vi "_MainOpenMV_New.vi"() -> (2 "Script Out":string)   [LabVIEW 2016]
uses:
  VIs/_subs/CameraSetup.ctl
panel:
  in  "Make Main":bool
  out "ROI":T1={"left"=0, "top"=0, "right"=320, "bottom"=240}
  in  "Set ROI":bool
  out "roi":string
  in  "Set Threshold":bool
  in  "clear":bool
  out "Plots":T2
  out "Lab":string="[10,90,-40,40,-40,40]"
  out "Tx Buffer":string
  in  "Play":bool
  in  "Serial Port":refnum<visa-resource-name>="ASRL30::INSTR"
  out "Version":string
  in  "Connect":bool
  out "FPS":dbl format="%#.2g"
  in  "Tabs":enum32{"Simple View", "REPL", "Python"}(tab)
  in  "Destination Info":enum32{"None", "UART", "SPI", "I2C", "WiFi"}(tab)
  in  "WiFi Info":T3={"WiFi"={"SSID"="", "Key"=""}, "SystemLink"={"APIKey"="", "Tag"="", "Type"="STRING"}}
  in  "Destination":enum16{"None", "UART", "SPI", "I2C", "WiFi"}(ring)
  out "Value":dbl(graph)
  in  "View":T4(ring)
  in  "Params":T5(tab)
  in  "Color Statistic":u16(ring) items=["l_mean", "l_median", "l_mode", "l_sdev", "l_min", "l_max", "l_lower quartile", "l_upper quartile", "a_mean", "a_median", "a_mode", "a_sdev", "a_min", "a_max", "a_lq", "a_uq", "b_mean", "b_median", "b_mode", "b_sdev", "b_max", "b_min", "b_lq", "b_uq", "All statistics"]
  in  "Gray Statistic":u16(ring)=1 items=["mean", "median", "mode", "sdev", "min", "max", "lower quartile", "upper quartile", "All statistics"]
  in  "Blob Params":T6={"B[0]_Feature"=enum."# blobs", "Lab thresholds"="[10,90,-20,20,-20,20]", "Min Pixels"=100, "Min Area (box)"=100, "Merge"=TRUE, "Margin for merge"=10}
  in  "Face Parameter":u16(ring) items=["# faces", "All data"]
  in  "QR Return":u16(ring)=4 items=["x", "y", "w", "h", "payload", "version", "ecc_level", "mask", "data_type", "All data"]
  in  "Ctrl D":bool
  in  "Grab Script":bool
  in  "Line":u8(slide) scale=0.0..25.0
  in  "Send Line":bool
  out "Console":string
  in  "Notepad":string
  in  "Ctrl C":bool
  out "rows":string="  1\n  2\n  3\n  4\n  5\n  6\n  7\n  8\n  9\n 10\n 11\n 12\n 13\n 14\n 15\n 16\n 17\n 18\n 19\n 20\n 21\n"
  in  "Script":string="# Show Color - lmean\n\nimport sensor, image, time\n\nsensor.reset()\nsensor.set_pixformat(sensor.RGB565)\nsensor.set_framesize(sensor.QVGA)\nsensor.skip_frames(time = 2000)\n\nsensor.set_auto_gain(False)\nsensor.set_auto_whitebal(False) \n\nclock = time.clock()\n\n\n\nwhile(True):\n    clock.tick()\n    img = sensor.snapshot()\n    \n    print(img.statistics()[0])\n"
  in  "New":bool
  in  "Load":bool
  in  "Save":bool
  in  "File":path
  in  "startCode":string
  out "Size":string
  in  "stop":bool
  out "image":picture
  # "LabVIEW OpenMV"
  # "Note: i2c and SPI and WiFi are having issues"
  # "Use P4 for Tx and P5 for Rx and GND for ground\n\nDefault BAUD rate is 19200 - you can change this\nby editing the Python code (Python tab)"
  # "Use P0 for MOSI, P1 for MISO, P2 for SCLK, P3 for SS (active low)\n and GND for ground\n\nThe default is being an SPI slave - note that you can miss data\nin this mode"
  # "Use P4 for SCL and P5 for SDA and GND for ground\n\nThis runs as an i2c slave"
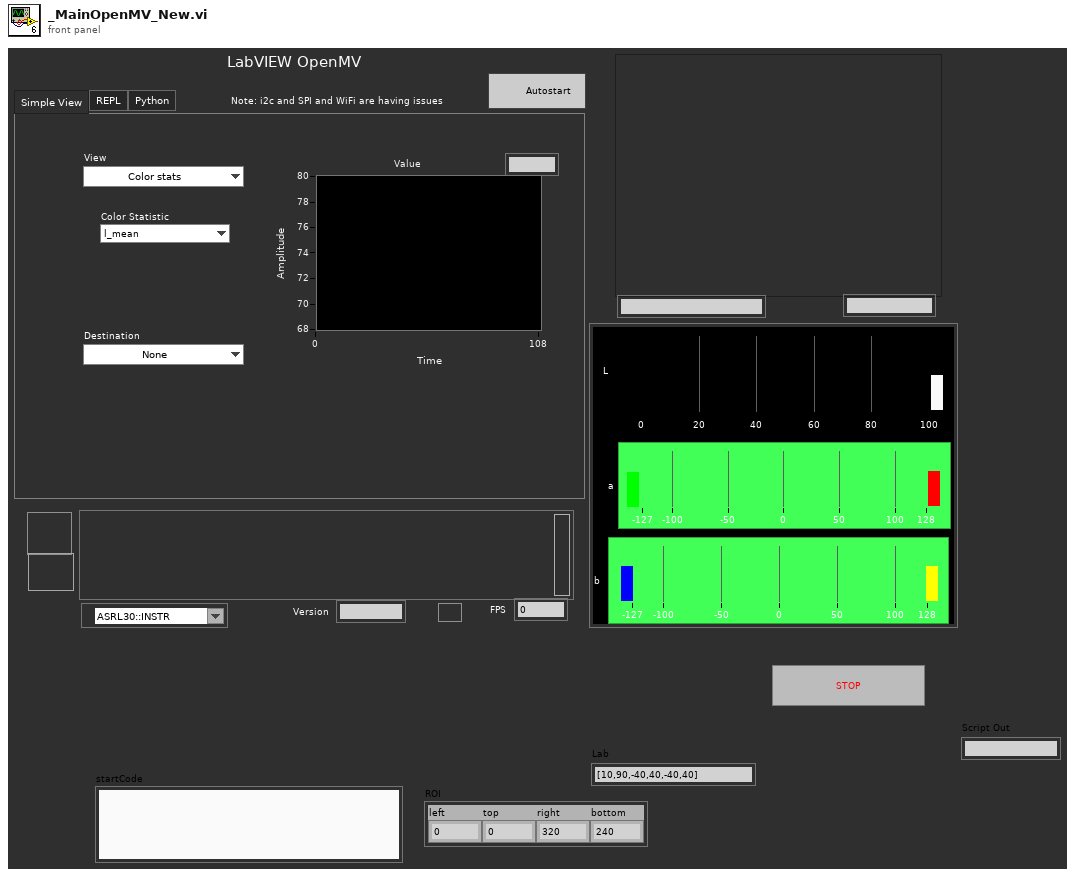
[diagram p1: front panel]
types:
  T1 = cluster{"left":i16, "top":i16, "right":i16, "bottom":i16}
  T2 = cluster{"L":dbl[], "a":cluster{i32, i32, dbl[]}, "b":cluster{i32, i32, dbl[]}}
  T3 = cluster{"WiFi":cluster{"SSID":string, "Key":string}, "SystemLink":cluster{"APIKey":string, "Tag":string, "Type":string}}
  T4 = enum16{"Color stats", "Greyscale stats", "Track Blobs", "Track Faces", "QRCode"}
  T5 = enum32{"C_ Stat", "G_Stats", "Blobs", "Face", "QR"}
  T6 = cluster{"B[0]_Feature":enum16{"x", "y", "width", "height", "pixels", "cx", "cy", "rotation", "code", "count", "# blobs", "All parameters"}, "Lab thresholds":string, "Min Pixels":i16, "Min Area (box)":i16, "Merge":bool, "Margin for merge":i16}
  T7 = enum8{"Enabled", "Disabled", "Disabled and Grayed Out"}
  T8 = typedef "CameraSetup.ctl" = cluster{"Format":enum16{"GRAYSCALE", "RGB565", "BAYER"}, "size":enum16{"QQQQVGA (40x30)", "QQQVGA (80x60)", "QQVGA (160x120)", "QVGA (320x240)", "VGA (640x480)", "LCD (128x160)", "B64x32 (64x32)", "B64x64", "B128x64", "B128x128"}, "Skip frames (ms)":u16, "autoGain":bool, "autoWhitebal":bool}
  T9 = typedef "imagedata.ctl" = cluster{"image type":i32, "image depth":i32, "image":u8[], "mask":u8[], "colors":u32[], "Rectangle":cluster{"left":i16, "top":i16, "right":i16, "bottom":i16}}
  T10 = cluster{"left":i32, "top":i32, "right":i32, "bottom":i32}
  T11 = typedef "eventvkey.ctl" = enum16{"ASCII", "Enter", "Return", "Shift", "Ctrl", "Alt", "Cmd", "Opt", "Caps", "NumLock", "Clear", "Break", "Up", "Down", "Left", "Right", "Insert", "Delete", "Home", "End", "PageUp", "PageDown", "Escape", "Help", "Pause", "ScrollLock", "F1", "F2", "F3", "F4", "F5", "F6", "F7", "F8", "F9", "F10", "F11", "F12", "F13", "F14", "F15", "F16", "F17", "F18", "F19", "F20", "F21", "F22", "F23", "F24", "Play", "VolumeUp", "VolumeDown", "Mute", "Two Byte Char"}
  T12 = cluster{"Shift":bool, "Ctrl":bool, "Alt":bool, "Cmd":bool, "Opt":bool}
  T13 = cluster{"Char":i16, "VKey":T11, "ScanCode":i16, "Mods":cluster{"Num Pad":bool, "Menu Key":bool}, "PlatMods":cluster{"Shift":bool, "Ctrl":bool, "Alt":bool, "Cmd":bool, "Opt":bool}, "FocusObj":refnum<vi>}
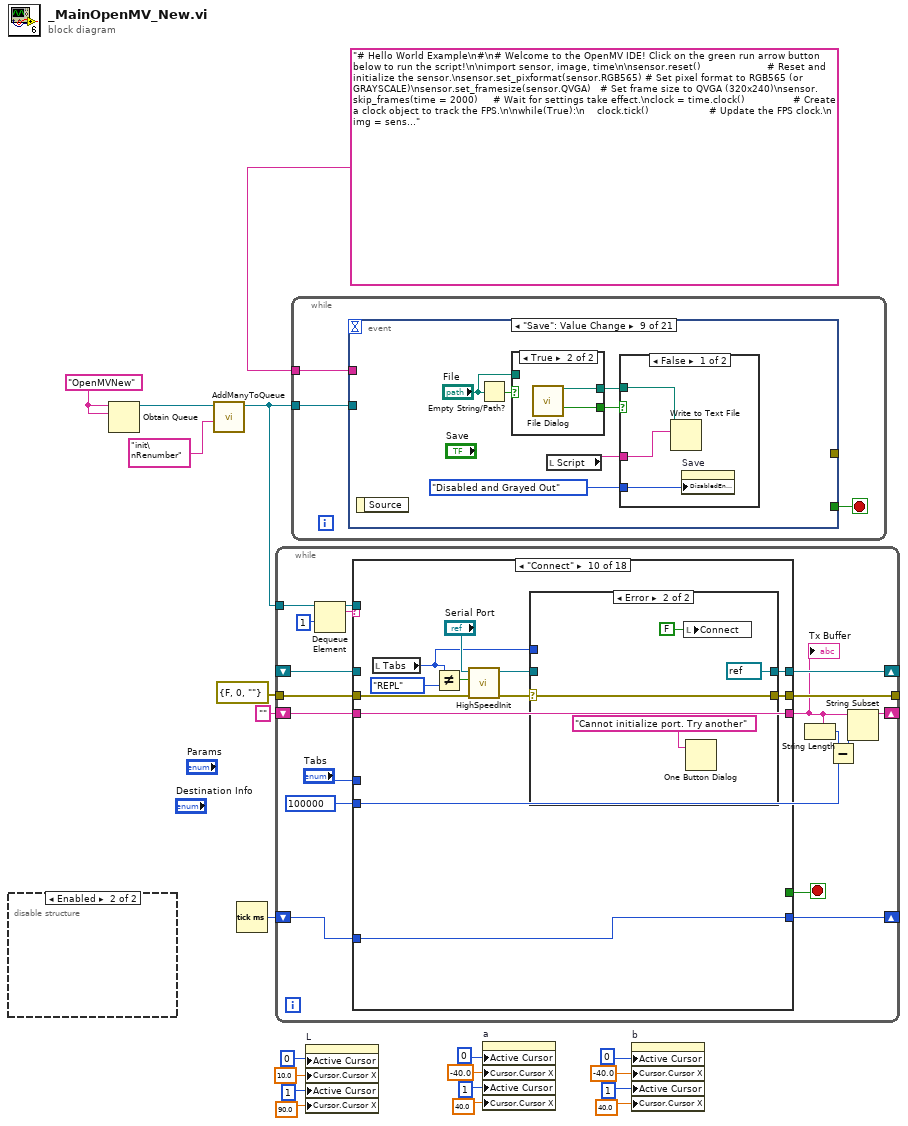
[diagram p0: block diagram]
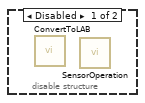
[diagram p2: hidden frame]
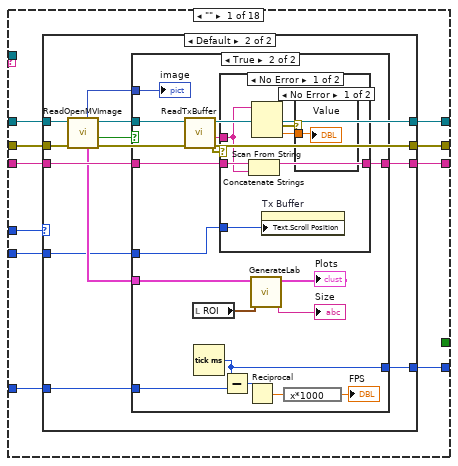
[diagram p3: hidden frame]
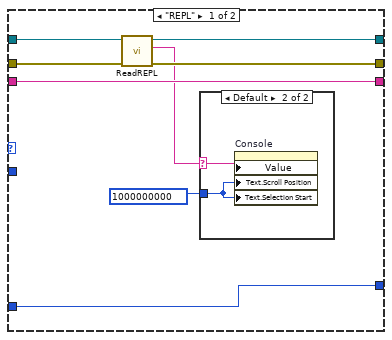
[diagram p4: hidden frame]
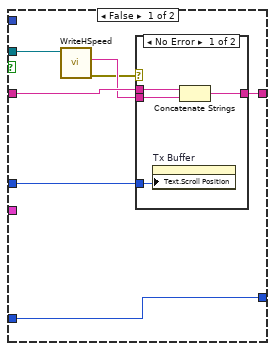
[diagram p6: hidden frame]
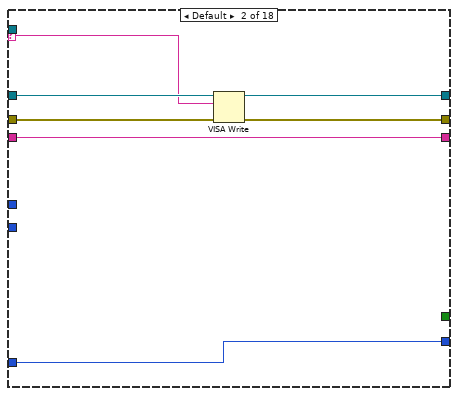
[diagram p10: hidden frame]
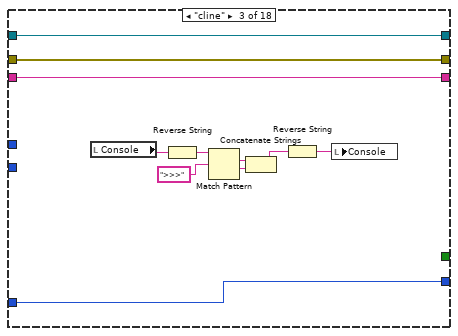
[diagram p11: hidden frame]
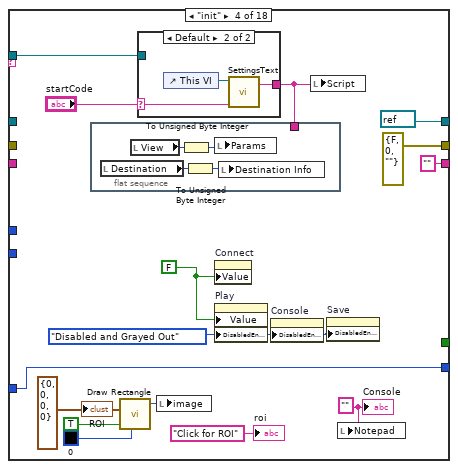
[diagram p12: hidden frame]
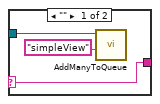
[diagram p13: hidden frame]
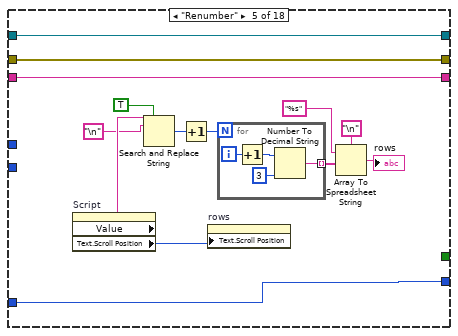
[diagram p14: hidden frame]
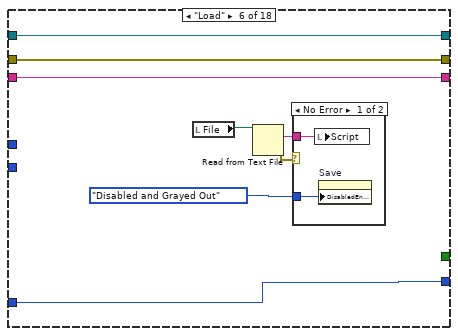
[diagram p15: hidden frame]
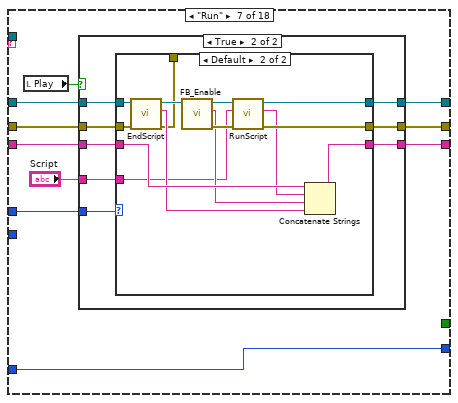
[diagram p17: hidden frame]
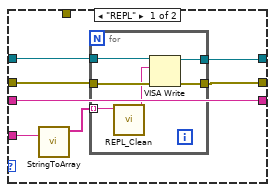
[diagram p19: hidden frame]
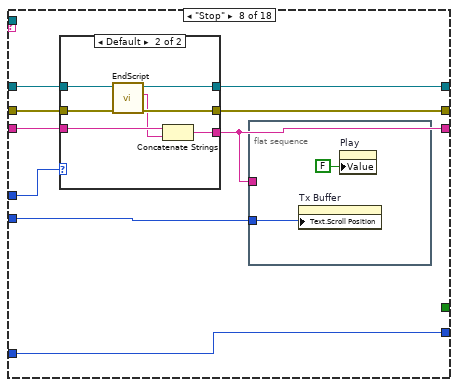
[diagram p20: hidden frame]
diagram:
  w20 = "OpenMVNew" ("name (unnamed)")
  n1 = disable-structure shown="Enabled" {
    frame Disabled {
      n2 = call "ConvertToLAB.vi"() -> ()  [unwired: 9 in, 3 out]
      n3 = call "SensorOperation.vi"() -> ()  [unwired: 11 in, 1 out]
    }
    frame Enabled {
    }
  }
  n4 = Obtain Queue(name (unnamed)=w20, element data type=w20) -> (queue out=w15:refnum<queue>)  [unwired: 3 in, 2 out]
  n5 = call "AddManyToQueue.vi"("Cmds"="init\nRenumber", "Queue in"=w15) -> ("Queue out"=w17:refnum<queue>)  [unwired: 9 in]
  n6 = Tick Count (ms)() -> (millisecond timer value=w18:u32)
  n7 = while {
    tunnel: w17 -> [w37]
    shift-right: [w34] -> _
    shift-left: _ -> [w35]
    shift-right: [w28] -> _
    shift-left: "" ("Tx Buffer") -> [w27]
    tunnel: errorcluster {"status"=FALSE, "code"=0, "source"=""} ("error out") -> [w32]
    tunnel: [w31] -> _
    shift-right: [w30] -> _
    shift-left: w18 -> [w29]
    stop <- w33 stop-if-true
    w25 = 100000 ("length (rest)")
    n8 = Dequeue Element(queue=w37, timeout in ms (-1)=1) -> (queue out=w21:refnum<queue>, element=w36:string)  [unwired: 1 in, 2 out]
    n9 = case shown="\"Connect\"" w36 {
      selector: w36 -> [_ w107 _ _ _ _ _ _ _ _ _ _ _ _ _ _ _ _]
      tunnel: w35 -> [w48 w111 w122 _ w163 w175 w187 w234 w258 _ w301 w318 w342 w350 w374 w422 w427 w435]
      tunnel: [w45 w108 w122 refnum<visa-resource-name> refnum ("VISA Refnum out") w163 w175 w185 w231 w255 w270 refnum<visa-resource-name> refnum ("VISA Refnum out") w318 w342 w350 w374 w422 w427 w435] -> w34
      tunnel: [w46 w109 w121 errorcluster {"status"=FALSE, "code"=0, "source"=""} ("error out") w162 w174 w184 w232 w256 w269 w299 w317 w341 w349 w373 w421 w428 w434] -> w31
      tunnel: w32 -> [w47 w110 w121 _ w162 w174 w186 w233 w257 w268 w300 w317 w341 w349 w373 w421 w428 w434]
      tunnel: w27 -> [w44 w113 w124 _ w161 w173 w183 w229 w253 w267 w303 w316 w340 w348 w376 _ w425 w433]
      tunnel: [w43 w113 w124 "" ("Tx Buffer") w161 w173 w182 w227 w251 w267 w303 w316 w340 w348 w376 "" ("Tx Buffer") w424 w433] -> w24
      tunnel: [_ _ _ _ _ _ _ _ _ _ _ _ _ _ _ _ _ TRUE] -> w33
      tunnel: [w42 w112 w123 w136 w160 w172 w181 w230 w254 w265 w297 w314 w339 w347 w375 w423 w429 w431] -> w30
      tunnel: w29 -> [w41 w112 w123 w136 w160 w172 w181 w230 w254 w265 w297 w314 w339 w347 w375 w423 w429 w431]
      tunnel: w25 -> [w40 _ _ _ _ _ _ w228 w252 _ w293 _ _ _ _ _ _ _]
      tunnel: "Tabs" -> [w39 _ _ _ _ _ w179 w226 _ _ _ _ _ _ _ _ _ _]
      tunnel: w21 -> [_ _ _ w125 _ _ _ _ _ _ _ _ _ _ _ _ _ _]
      frame "" {
        n10 = case shown="Default" w39 {
          tunnel: w48 -> [w56 w68]
          tunnel: w47 -> [w55 w67]
          tunnel: [w53 w66] -> w46
          tunnel: [w54 w65] -> w45
          tunnel: w44 -> [w52 w64]
          tunnel: [w52 w63] -> w43
          tunnel: [w51 w62] -> w42
          tunnel: w41 -> [w51 w61]
          tunnel: w40 -> [_ w59]
          frame "REPL" {
            n11 = call "ReadREPL.vi"("error in (no error)"=w55, "VISA Refnum in"=w56) -> ("error out"=w53:errorcluster, "String"=w49:string, "VISA Refnum out"=w54:refnum<visa-resource-name>)  [unwired: 6 in, 1 out]
            n12 = case shown="Default" w49 {
              selector: w49 -> [_ w57]
              tunnel: u32 1000000000 ("Text.Selection:Start") -> [_ w58]
              frame "" {
              }
              frame Default {
                n13 = property on="Console" class="Str"("Value"=w57, "Text.Scroll Position"=w58, "Text.Selection Start"=w58) -> ()  [unwired: 2 in, 2 out]
              }
            }
          }
          frame Default {
            n14 = call "ReadOpenMVImage.vi"("error in"=w67, "VISA Refnum in"=w68) -> ("error out"=w66:errorcluster, "Good?"=w70:bool, "VISA Refnum out"=w65:refnum<visa-resource-name>, "image data"=w60:T9, "new picture"=w69:picture)  [unwired: 4 in, 1 out]
            n15 = case shown="True" w70 {
              tunnel: w69 -> [_ w92]
              tunnel: w65 -> [w73 w98]
              tunnel: [w75 w88] -> w63
              tunnel: w64 -> [w76 w86]
              tunnel: [w77 w97] -> w62
              tunnel: w61 -> [w77 w96]
              tunnel: w60 -> [_ w90]
              tunnel: w59 -> [w74 w83]
              frame False {
                n16 = call "WriteHSpeed.vi"("VISA Refnum in"=w73) -> ("error out"=w71:errorcluster, "read buffer"=w72:string)  [unwired: 8 in, 1 out]
                n17 = case shown="No Error" w71 {
                  tunnel: w72 -> [w81 _]
                  tunnel: w76 -> [w80 w82]
                  tunnel: [w79 w82] -> w75
                  tunnel: w74 -> [w78 _]
                  frame No Error {
                    n18 = property on="Tx Buffer" class="Str"("Text.Scroll Position"=w78) -> ()  [unwired: 2 in, 2 out]
                    n19 = Concatenate Strings(w80, w81) -> (w79:string)
                  }
                  frame Error {
                  }
                }
              }
              frame True {
                n20 = call "ReadTxBuffer.vi"("VISA Refnum in"=w98) -> ("error out"=w84:errorcluster, "Tx Buffer"=w85:string)  [unwired: 7 in, 2 out]
                n21 = local read "ROI"() -> (w89:T1)
                n22 = Tick Count (ms)() -> (millisecond timer value=w97:u32)
                n23 = case shown="No Error" w84 {
                  tunnel: [w104 w106] -> w88
                  tunnel: w86 -> [w101 w106]
                  tunnel: w85 -> [w100 _]
                  tunnel: w83 -> [w99 _]
                  frame No Error {
                    n24 = Concatenate Strings(w101, w100) -> (w104:string)
                    n25 = Scan From String(input string=w100) -> (error out=w103:errorcluster, output 1=w102:dbl)  [unwired: 4 in, 2 out]
                    n26 = property on="Tx Buffer" class="Str"("Text.Scroll Position"=w99) -> ()  [unwired: 2 in, 2 out]
                    n27 = case shown="No Error" w103 {
                      tunnel: w102 -> [w105 _]
                      frame No Error {
                        "Value" <- w105
                      }
                      frame Error {
                      }
                    }
                  }
                  frame Error {
                  }
                }
                n28 = Subtract(x=w97, y=w96) -> (x-y=w93:u32)
                n29 = Reciprocal(x=w93) -> (1/x=w95:dbl)
                n30 = call "GenerateLab.vi"("ROI"=w89, "image data"=w90) -> ("Dimensions"=→"Size":string, "Plots"=→"Plots":T2)  [unwired: 8 in]
                n31 = expression code="x*1000"(w95) -> (→"FPS":dbl)
                "image" <- w92
              }
            }
          }
        }
      }
      frame Default {
        n32 = VISA Write(VISA resource name=w111, write buffer=w107, error in (no error)=w110) -> (VISA resource name out=w108:refnum<visa-resource-name>, error out=w109:errorcluster)  [unwired: 1 out]
      }
      frame "cline" {
        n33 = local read "Console"() -> (w114:string)
        n34 = Reverse String(1:w114) -> (0:w120:string)
        n35 = Match Pattern(string=w120, regular expression=">>>") -> (match substring=w117:string, after substring=w118:string)  [unwired: 1 in, 2 out]
        n36 = Concatenate Strings(w117, w118) -> (w116:string)
        n37 = Reverse String(1:w116) -> (0:w115:string)
        n38 = local write "Console"(w115) -> ()
      }
      frame "init" {
        w131 = "" ("Tx Buffer")
        w129 = T1 {"left"=0, "top"=0, "right"=0, "bottom"=0} ("rect")
        w130 = T7."Disabled and Grayed Out" ("Disabled")
        w132 = FALSE ("Connect")
        n39 = flat-sequence {
          tunnel: w126 -> [_]
          frame #0 {
            n40 = local read "Destination"() -> (w146:enum16{"None", "UART", "SPI", "I2C", "WiFi"})
            n41 = local read "View"() -> (w149:T4)
            n42 = To Unsigned Byte Integer(number=w149) -> (unsigned 8bit integer=w148:u8)
            n43 = To Unsigned Byte Integer(number=w146) -> (unsigned 8bit integer=w147:u8)
            n44 = local write "Params"(w148) -> ()
            n45 = local write "Destination Info"(w147) -> ()
          }
        }
        n46 = call <vilib>:"Draw Rectangle.vi"("rect"=w129, "fill?(F)"=TRUE, "color(black)"=u32 0) -> ("new picture"=w133:picture)  [unwired: 6 in]
        n47 = case shown="Default" "startCode" {
          selector: "startCode" -> [w142 w143]
          tunnel: [w142 w144] -> w126
          tunnel: w125 -> [w141 _]
          frame "" {
            n48 = call "AddManyToQueue.vi"("Cmds"="simpleView", "Queue in"=w141) -> ()  [unwired: 9 in, 1 out]
          }
          frame Default {
            n49 = control-ref of="This VI"() -> (w145:refnum<vi>)
            n50 = call "SettingsText.vi"("Saved code"=w143, "VI in"=w145) -> ("Python Code out"=w144:string)  [unwired: 8 in, 1 out]
          }
        }
        n51 = local write "image"(w133) -> ()
        n52 = property on="Connect" class="Bool (strict)"("Value"=w132) -> ()  [unwired: 2 in, 2 out]
        n53 = property on="Play" class="Bool (strict)"("Value"=w132, "DisabledEnum"=w130) -> ()  [unwired: 2 in, 2 out]
        n54 = property on="Console" class="Str"("DisabledEnum"=w130) -> ()  [unwired: 2 in, 2 out]
        n55 = local write "Script"(w126) -> ()
        n56 = property on="Save" class="Bool"("DisabledEnum"=w130) -> ()  [unwired: 2 in, 2 out]
        n57 = local write "Notepad"(w131) -> ()
        "Console" <- w131
        "roi" <- "Click for ROI" ("roi")
        "ROI" <- w129
      }
      frame "Renumber" {
        n58 = property on="Script" class="Str"() -> ("Value"=w159:string, "Text.Scroll Position"=w158:u32)  [unwired: 2 in, 2 out]
        n59 = Search and Replace String(replace all?=TRUE ("replace all? (F)"), input string=w159, search string="\n") -> (number of replacements=w157:i32)  [unwired: 5 in, 3 out]
        n60 = Increment(x=w157) -> (x+1=w150:i32)
        n61 = property on="rows" class="Str"("Text.Scroll Position"=w158) -> ()  [unwired: 2 in, 2 out]
        n62 = for {
          N: w150 -> [_]
          tunnel: [w167] -> w155 mode=indexing
          i -> [w164]
          n63 = Increment(x=w164) -> (x+1=w166:i32)
          n64 = Number To Decimal String(number=w166, width (-)=i16 3) -> (decimal integer string=w167:string)
        }
        n65 = Array To Spreadsheet String(delimiter (Tab)="\n", array=w155, 3:"%s" ("format string")) -> (spreadsheet string=→"rows":string)
      }
      frame "Load" {
        n66 = local read "File"() -> (w171:path)
        n67 = Read from Text File(file (use dialog)=w171) -> (text=w168:string, error out=w169:errorcluster)  [unwired: 3 in, 2 out]
        n68 = case shown="No Error" w169 {
          tunnel: T7."Disabled and Grayed Out" ("Disabled") -> [w177 _]
          tunnel: w168 -> [w176 _]
          frame No Error {
            n69 = local write "Script"(w176) -> ()
            n70 = property on="Save" class="Bool"("DisabledEnum"=w177) -> ()  [unwired: 2 in, 2 out]
          }
          frame Error {
          }
        }
      }
      frame "Run" {
        n71 = local read "Play"() -> (w180:bool)
        n72 = case shown="True" w180 {
          tunnel: w187 -> [w190 w198]
          tunnel: w186 -> [w189 w197]
          tunnel: [w190 w196] -> w185
          tunnel: [w189 w195] -> w184
          tunnel: w183 -> [w188 w193]
          tunnel: [w188 w194] -> w182
          tunnel: w179 -> [_ w192]
          tunnel: "Script" -> [_ w191]
          frame False {
          }
          frame True {
            n73 = case shown="Default" w192 {
              tunnel: w198 -> [w204 w222]
              tunnel: w197 -> [w203 w221]
              tunnel: [w201 w220] -> w196
              tunnel: [w202 w219] -> w195
              tunnel: [w199 w218] -> w194
              tunnel: w193 -> [w199 w217]
              tunnel: w191 -> [w200 w213]
              tunnel: [_ w212] -> _
              frame "REPL" {
                n74 = call "StringToArray.vi"("write buffer"=w200) -> ("Array"=w205:string[])  [unwired: 10 in]
                n75 = for {
                  tunnel: w205 -> [w207] mode=indexing
                  tunnel: w204 -> [w211]
                  tunnel: w203 -> [w210]
                  tunnel: [w209] -> w202
                  tunnel: [w208] -> w201
                  n76 = call "REPL_Clean.vi"("Code in"=w207) -> ("Code cleaned"=w206:string)  [unwired: 10 in]
                  n77 = VISA Write(VISA resource name=w211, write buffer=w206, error in (no error)=w210) -> (VISA resource name out=w208:refnum<visa-resource-name>, error out=w209:errorcluster)  [unwired: 1 out]
                }
              }
              frame Default {
                n78 = call "EndScript.vi"("error in (no error)"=w221, "VISA Refnum in"=w222) -> ("error out"=w212:errorcluster, "Tx for stopping code"=w214:string, "VISA Refnum out"=w225:refnum<visa-resource-name>)  [unwired: 7 in]
                n79 = call "FB_Enable.vi"("VISA Refnum in"=w225) -> ("error out"=w224:errorcluster, "Reply"=w215:string, "VISA Refnum out"=w223:refnum<visa-resource-name>)  [unwired: 8 in]
                n80 = call "RunScript.vi"("error in"=w224, "script"=w213, "VISA Refnum in"=w223) -> ("error out"=w219:errorcluster, "Tx"=w216:string, "VISA Refnum out"=w220:refnum<visa-resource-name>)  [unwired: 6 in]
                n81 = Concatenate Strings(w217, w216, w215, w214) -> (w218:string)
              }
            }
          }
        }
      }
      frame "Stop" {
        n82 = case shown="Default" w226 {
          tunnel: w234 -> [w238 w247]
          tunnel: w233 -> [w236 w246]
          tunnel: [w235 w245] -> w232
          tunnel: [w237 w244] -> w231
          tunnel: w229 -> [w240 w243]
          tunnel: [w240 w241] -> w227
          frame "REPL" {
            n83 = VISA Write(VISA resource name=w238, write buffer="\u0003", error in (no error)=w236) -> (VISA resource name out=w237:refnum<visa-resource-name>, error out=w235:errorcluster)  [unwired: 1 out]
          }
          frame Default {
            n84 = call "EndScript.vi"("error in (no error)"=w246, "VISA Refnum in"=w247) -> ("error out"=w245:errorcluster, "Tx for stopping code"=w242:string, "VISA Refnum out"=w244:refnum<visa-resource-name>)  [unwired: 7 in]
            n85 = Concatenate Strings(w243, w242) -> (w241:string)
          }
        }
        n86 = flat-sequence {
          tunnel: w228 -> [w249]
          tunnel: w227 -> [_]
          frame #0 {
            n87 = property on="Tx Buffer" class="Str"("Text.Scroll Position"=w249) -> ()  [unwired: 2 in, 2 out]
            n88 = property on="Play" class="Bool (strict)"("Value"=FALSE ("Play")) -> ()  [unwired: 2 in, 2 out]
          }
        }
      }
      frame "stopForREPL" {
        n89 = call "EndScript.vi"("error in (no error)"=w257, "VISA Refnum in"=w258) -> ("error out"=w256:errorcluster, "Tx for stopping code"=w250:string, "VISA Refnum out"=w255:refnum<visa-resource-name>)  [unwired: 7 in]
        n90 = Concatenate Strings(w253, w250) -> (w251:string)
        n91 = flat-sequence {
          tunnel: w252 -> [w260]
          tunnel: w251 -> [_]
          frame #0 {
            n92 = property on="Tx Buffer" class="Str"("Text.Scroll Position"=w260) -> ()  [unwired: 2 in, 2 out]
            n93 = property on="Play" class="Bool (strict)"("Value"=FALSE ("Play")) -> ()  [unwired: 2 in, 2 out]
          }
        }
      }
      frame "Connect" {
        n94 = local read "Tabs"() -> (w262:enum32{"Simple View", "REPL", "Python"})
        n95 = Not Equal?(x=w262, y=enum32{"Simple View", "REPL", "Python"}."REPL") -> (x != y?=w264:bool)
        n96 = call "HighSpeedInit.vi"("error in"=w268, "Fast"=w264, "VISA Refnum in"="Serial Port") -> ("error out"=w261:errorcluster, "VISA Refnum out"=w271:refnum<visa-resource-name>)  [unwired: 7 in]
        n97 = case shown="Error" w261 {
          selector: w261 -> [w272 w291]
          tunnel: w271 -> [w277 _]
          tunnel: [w276 refnum<visa-resource-name> refnum ("VISA Refnum out")] -> w270
          tunnel: [w275 w291] -> w269
          tunnel: w262 -> [w274 _]
          frame No Error {
            w273 = T7."Enabled" ("Disabled")
            n98 = property on="Play" class="Bool (strict)"("DisabledEnum"=w273) -> ()  [unwired: 2 in, 2 out]
            n99 = case shown="\"REPL\"" w274 {
              tunnel: w272 -> [w281 w288]
              tunnel: w277 -> [w283 w287]
              tunnel: [w279 w285] -> w276
              tunnel: [w280 w284] -> w275
              tunnel: w273 -> [w278 _]
              frame "REPL" {
                n100 = property on="Console" class="Str"("DisabledEnum"=w278) -> ()  [unwired: 2 in, 2 out]
                n101 = VISA Write(VISA resource name=w283, write buffer="\n\n", error in (no error)=w281) -> (VISA resource name out=w279:refnum<visa-resource-name>, error out=w280:errorcluster)  [unwired: 1 out]
              }
              frame Default {
                n102 = call "AskVersion.vi"("error in"=w288, "VISA Refnum in"=w287) -> ("error out"=w284:errorcluster, "Version"=→"Version":string, "VISA Refnum out"=w285:refnum<visa-resource-name>)  [unwired: 7 in]
              }
            }
          }
          frame Error {
            n103 = local write "Connect"(FALSE ("Connect")) -> ()
            n104 = One Button Dialog(message="Cannot initialize port. Try another") -> ()  [unwired: 1 in, 1 out]
          }
        }
      }
      frame "Disconnect" {
        w294 = T7."Disabled and Grayed Out" ("Disabled")
        n105 = local read "Tabs"() -> (w295:enum32{"Simple View", "REPL", "Python"})
        n106 = property on="Tx Buffer" class="Str"("Text.Scroll Position"=w293) -> ()  [unwired: 2 in, 2 out]
        n107 = case shown="Default" w295 {
          tunnel: [w306 w310] -> w302
          tunnel: w301 -> [w306 w309]
          tunnel: w300 -> [w305 w308]
          tunnel: [w305 w307] -> w299
          frame "REPL" {
          }
          frame Default {
            n108 = call "EndScript.vi"("error in (no error)"=w308, "VISA Refnum in"=w309) -> ("error out"=w307:errorcluster, "VISA Refnum out"=w310:refnum<visa-resource-name>)  [unwired: 7 in, 1 out]
          }
        }
        n109 = call "CloseHS.vi"("error in (no error)"=w299, "VISA Refnum in"=w302) -> ()  [unwired: 10 in]
        n110 = local write "Connect"(FALSE ("Connect")) -> ()
        n111 = property on="Play" class="Bool (strict)"("Value"=FALSE ("Play"), "DisabledEnum"=w294) -> ()  [unwired: 2 in, 2 out]
        n112 = property on="Console" class="Str"("DisabledEnum"=w294) -> ()  [unwired: 2 in, 2 out]
      }
      frame "ROI" {
        n113 = local read "image"() -> (w315:picture)
        n114 = local read "ROI"() -> (w311:T1)
        n115 = call "OpenMV_SelectROI.vi"("ROI"=w311, "image"=w315) -> ("Rect"=w313:T10)  [unwired: 1 in]
        n116 = local write "ROI"(w313) -> ()
        n117 = call "ROIText.vi"("ROI"=w313) -> ("r"=w312:string)  [unwired: 7 in, 3 out]
        n118 = local write "roi"(w312) -> ()
      }
      frame "Lab" {
        n119 = property on="L" class="WFGraph (strict)"("Active Cursor"=u32 0, "Active Cursor"=u32 1) -> ("Cursor.Cursor X"=w332:dbl, "Cursor.Cursor X"=w331:dbl)  [unwired: 2 in, 2 out]
        n120 = property on="a" class="WFGraph (strict)"("Active Cursor"=u32 0, "Active Cursor"=u32 1) -> ("Cursor.Cursor X"=w333:dbl, "Cursor.Cursor X"=w334:dbl)  [unwired: 2 in, 2 out]
        n121 = property on="b" class="WFGraph (strict)"("Active Cursor"=u32 0, "Active Cursor"=u32 1) -> ("Cursor.Cursor X"=w335:dbl, "Cursor.Cursor X"=w336:dbl)  [unwired: 2 in, 2 out]
        n122 = Max & Min(x=w332, y=w331) -> (max(x,y)=w324:dbl, min(x,y)=w323:dbl)
        n123 = Max & Min(x=w333, y=w334) -> (max(x,y)=w322:dbl, min(x,y)=w321:dbl)
        n124 = Max & Min(x=w335, y=w336) -> (max(x,y)=w319:dbl, min(x,y)=w320:dbl)
        n125 = Format Into String(format string="[%d,%d,%d,%d,%d,%d]", w323, w324, w321, w322, w320, w319) -> (resulting string=→"Lab":string)  [unwired: 2 in, 1 out]
      }
      frame "LabPopup" {
        n126 = local read "image"() -> (w345:picture)
        n127 = local read "ROI"() -> (w343:T1)
        n128 = call "OpenMV_SelectLab.vi"("ROI"=w343, "image"=w345) -> ("ROI out"=w344:T10, "thresholds"=w346:dbl[])
        n129 = for {
          tunnel: w346 -> [w351] mode=indexing
          i -> [w355]
          n130 = Quotient & Remainder(x=w355, y=2) -> (x-y*floor(x/y)=w352:i32, floor(x/y)=w353:i32)
          n131 = case shown="0" w353 {
            tunnel: w352 -> [_ w357 w359 w361]
            tunnel: w351 -> [_ w356 w358 w360]
            frame Default {
            }
            frame 0 {
              n132 = property on="L" class="WFGraph (strict)"("Active Cursor"=w357, "Cursor.Cursor X"=w356) -> ()  [unwired: 2 in, 2 out]
            }
            frame 1 {
              n133 = property on="a" class="WFGraph (strict)"("Active Cursor"=w359, "Cursor.Cursor X"=w358) -> ()  [unwired: 2 in, 2 out]
            }
            frame 2 {
              n134 = property on="b" class="WFGraph (strict)"("Active Cursor"=w361, "Cursor.Cursor X"=w360) -> ()  [unwired: 2 in, 2 out]
            }
          }
        }
        n135 = local write "ROI"(w344) -> ()
      }
      frame "simpleView" {
        n136 = local read "Lab"() -> (w367:string)
        n137 = local read "ROI"() -> (w368:T1)
        n138 = case shown="\"Greyscale stats\"" "View" {
          tunnel: "Destination" -> [w383 w394 w403 w410 w417]
          tunnel: [w382 w393 w402 w408 w415] -> w365
          tunnel: "WiFi Info" -> [w381 w392 w401 w409 w416]
          tunnel: w368 -> [w380 w391 w396 w406 w413]
          tunnel: w367 -> [_ _ w398 _ _]
          tunnel: [w379 w390 w397 w407 w414] -> _
          frame "Color stats", Default {
            n139 = call "simpleStatistics.vi"("WiFi Info"=w381, "ROI"=w380, "Output"=w383, "Camera Setup"=T8 {"Format"=enum."RGB565", "size"=enum."QVGA (320x240)", "Skip frames (ms)"=2000, "autoGain"=TRUE, "autoWhitebal"=TRUE}, "Statistic"="Color Statistic") -> ("error out"=w379:errorcluster, "Python Code"=w382:string)  [unwired: 4 in, 1 out]
          }
          frame "Greyscale stats" {
            n140 = Not Equal?(x="Gray Statistic", y=u8 8) -> (x != y?=w388:bool)
            n141 = Select(t="Gray Statistic", s=w388, f=u8 24 ("y")) -> (s? t:f=w387:u16)
            n142 = call "simpleStatistics.vi"("WiFi Info"=w392, "ROI"=w391, "Output"=w394, "Camera Setup"=T8 {"Format"=enum."GRAYSCALE", "size"=enum."QVGA (320x240)", "Skip frames (ms)"=2000, "autoGain"=TRUE, "autoWhitebal"=TRUE}, "Statistic"=w387) -> ("error out"=w390:errorcluster, "Python Code"=w393:string)  [unwired: 4 in, 1 out]
          }
          frame "Track Blobs" {
            n143 = Bundle By Name(cluster="Blob Params", "Lab thresholds"=w398) -> (w399:T6)
            n144 = call "trackBlobs.vi"("WiFi Info"=w401, "ROI"=w396, "Output"=w403, "Camera Setup"=T8 {"Format"=enum."RGB565", "size"=enum."QVGA (320x240)", "Skip frames (ms)"=2000, "autoGain"=TRUE, "autoWhitebal"=TRUE}, "Blob Params"=w399) -> ("error out"=w397:errorcluster, "Python Code"=w402:string)  [unwired: 4 in, 1 out]
          }
          frame "QRCode" {
            n145 = call "QRCodes.vi"("WiFi Info"=w409, "ROI"=w406, "Output"=w410, "Camera Setup"=T8 {"Format"=enum."RGB565", "size"=enum."QVGA (320x240)", "Skip frames (ms)"=2000, "autoGain"=FALSE, "autoWhitebal"=FALSE}, "Value"="QR Return") -> ("error out"=w407:errorcluster, "Python Code"=w408:string)  [unwired: 4 in, 1 out]
          }
          frame "Track Faces" {
            n146 = call "trackFaces.vi"("WiFi Info"=w416, "ROI"=w413, "Output"=w417, "Camera Setup"=T8 {"Format"=enum."GRAYSCALE", "size"=enum."QVGA (320x240)", "Skip frames (ms)"=2000, "autoGain"=FALSE, "autoWhitebal"=FALSE}, "Value"="Face Parameter") -> ("error out"=w414:errorcluster, "Python Code"=w415:string)  [unwired: 4 in, 1 out]
          }
        }
        n147 = Equal?(x=T4."Track Blobs" ("View"), y="View") -> (x = y?=w372:bool)
        n148 = for {
          N: 2 -> [_]
          tunnel: w372 -> [w419]
          i -> [w418]
          n149 = property on="L" class="WFGraph (strict)"("Active Cursor"=w418, "Cursor.Visible"=w419) -> ()  [unwired: 2 in, 2 out]
          n150 = property on="a" class="WFGraph (strict)"("Active Cursor"=w418, "Cursor.Visible"=w419) -> ()  [unwired: 2 in, 2 out]
          n151 = property on="b" class="WFGraph (strict)"("Active Cursor"=w418, "Cursor.Visible"=w419) -> ()  [unwired: 2 in, 2 out]
        }
        n152 = control-ref of="This VI"() -> (w364:refnum<vi>)
        n153 = call "SettingsText.vi"("Python Code in"=w365, "VI in"=w364) -> ("Python Code out"=w362:string)  [unwired: 8 in, 1 out]
        n154 = local write "Script"(w362) -> ()
      }
      frame "Clear" {
      }
      frame "Main.py" {
        n155 = local read "Script"() -> (w426:string)
        n156 = call "OMV_UploadMainPY.vi"("Script"=w426, "Tx Buffer"=w425, "VISA Refnum in"=w427) -> ("Tx Buffer Out"=w424:string)  [unwired: 8 in]
      }
      frame "Done" {
        n157 = local read "Script"() -> (→"Script Out":string)
      }
    }
    "Tx Buffer" <- w24
    n158 = String Length(string=w24) -> (length=w26:i32)
    n159 = Subtract(x=w26, y=w25) -> (x-y=w23:i32)
    n160 = String Subset(string=w24, offset (0)=w23) -> (substring=w28:string)  [unwired: 1 in]
  }
  n161 = while {
    tunnel: w17 -> [w437]
    tunnel: "# Hello World Example\n#\n# Welcome to the OpenMV IDE! Click on the green run arrow button below to run the script!\n\nimport sensor, image, time\n\nsensor.reset()                      # Reset and initialize the sensor.\nsensor.set_pixformat(sensor.RGB565) # Set pixel format to RGB565 (or GRAYSCALE)\nsensor.set_framesize(sensor.QVGA)   # Set frame size to QVGA (320x240)\nsensor.skip_frames(time = 2000)     # Wait for settings take effect.\nclock = time.clock()                # Create a clock object to track the FPS.\n\nwhile(True):\n    clock.tick()                    # Update the FPS clock.\n    img = sensor.snapshot()         # Take a picture and return the image.\n    print(clock.fps())              # Note: OpenMV Cam runs about half as fast when connected\n                                    # to the IDE. The FPS should increase once disconnected.\n" ("startCode") -> [w436]
    stop <- w438 stop-if-true
    n162 = event shown="[8] \"Save\": Value Change" {
      selector: _ -> [_ _ _ _ _ _ _ _ _ _ _ _ _ _ _ _ _ _ _ _ _]
      dyn-events: _ -> [_ _ _ _ _ _ _ _ _ _ _ _ _ _ _ _ _ _ _ _ _]
      timeout: _ -> [_ _ _ _ _ _ _ _ _ _ _ _ _ _ _ _ _ _ _ _ _]
      tunnel: [_ "stop" _ _ _ _ _ _ _ _ _ _ _ _ _ _ _ _ _ _ _] -> w438
      tunnel: w437 -> [_ w441 w451 w460 w465 w467 _ w475 _ w499 w506 w510 w513 w516 _ _ _ w534 _ w539 w545]
      tunnel: w436 -> [_ _ _ _ _ _ w471 _ _ _ _ _ _ _ _ _ _ _ _ _ _]
      tunnel: [_ _ _ _ _ _ _ _ _ _ _ _ _ _ w518 w521 _ _ _ _ _] -> _
      event Timeout {
        n163 = event-data() -> ()  [unwired: 1 in, 1 out]
      }
      event "stop": Value Change {
        n164 = event-data() -> ()  [unwired: 1 in, 1 out]
        n165 = local read "Connect"() -> (w439:bool)
        n166 = case shown="True" w439 {
          tunnel: w441 -> [w444 w447]
          tunnel: [w444 w446] -> w440
          frame False {
          }
          frame True {
            n167 = Enqueue Element(queue=w447, element="Disconnect") -> (queue out=w446:refnum<queue>)  [unwired: 2 in, 2 out]
          }
        }
        n168 = Enqueue Element(queue=w440, element="Done") -> ()  [unwired: 2 in, 3 out]
      }
      event "Tabs": Value Change {
        n169 = event-data() -> ("NewVal"=w448:enum32{"Simple View", "REPL", "Python"})  [unwired: 1 in]
        n170 = case shown="\"REPL\"" w448 {
          tunnel: w451 -> [w452 w454]
          tunnel: [w452 w453] -> w450
          frame Default {
          }
          frame "REPL" {
            n171 = call "AddManyToQueue.vi"("Cmds"="stopForREPL\nDisconnect", "Queue in"=w454) -> ("Queue out"=w453:refnum<queue>)  [unwired: 9 in]
          }
        }
        n172 = Enqueue Element(queue=w450, element="Renumber") -> ()  [unwired: 2 in, 3 out]
      }
      event "Play": Value Change {
        n173 = event-data() -> ()  [unwired: 1 in, 1 out]
        n174 = Select(t="Run" ("element"), s="Play", f="Stop" ("element")) -> (s? t:f=w456:string)
        n175 = Enqueue Element(queue=w460, element=w456) -> ()  [unwired: 2 in, 3 out]
      }
      event "Connect": Value Change {
        n176 = event-data() -> ()  [unwired: 1 in, 1 out]
        n177 = Select(t="Connect" ("element"), s="Connect", f="Disconnect" ("element")) -> (s? t:f=w463:string)
        n178 = Enqueue Element(queue=w465, element=w463) -> ()  [unwired: 2 in, 3 out]
      }
      event "Script": Value Change {
        n179 = event-data() -> ()  [unwired: 1 in, 1 out]
        n180 = Enqueue Element(queue=w467, element="Renumber") -> ()  [unwired: 2 in, 3 out]
        n181 = property on="Save" class="Bool"("DisabledEnum"=T7."Enabled" ("Disabled")) -> ()  [unwired: 2 in, 2 out]
      }
      event "New": Value Change {
        n182 = event-data() -> ()  [unwired: 1 in, 1 out]
        n183 = property on="Save" class="Bool"() -> ("DisabledEnum"=w470:T7)  [unwired: 2 in, 2 out]
        n184 = call "CheckReplace.vi"("DisabledEnum"=w470) -> ("Replace?"=w469:bool)  [unwired: 10 in]
        n185 = case shown="True" w469 {
          tunnel: w471 -> [_ w473]
          frame False {
          }
          frame True {
            n186 = property on="Save" class="Bool"("DisabledEnum"=T7."Enabled" ("Disabled")) -> ()  [unwired: 2 in, 2 out]
            n187 = local write "Script"(w473) -> ()
            n188 = local write "File"(path "" ("File")) -> ()
          }
        }
      }
      event "Load", "File": Value Change {
        n189 = event-data() -> ()  [unwired: 1 in, 1 out]
        n190 = property on="Save" class="Bool"() -> ("DisabledEnum"=w477:T7)  [unwired: 2 in, 2 out]
        n191 = call "CheckReplace.vi"("DisabledEnum"=w477) -> ("Replace?"=w476:bool)  [unwired: 10 in]
        n192 = case shown="True" w476 {
          tunnel: w475 -> [_ w480]
          frame False {
          }
          frame True {
            n193 = call "File Dialog2"() -> ("selected path"=w478:path, "cancelled"=w479:bool)  [unwired: 12 in, 2 out]
            n194 = case shown="False" w479 {
              tunnel: w480 -> [w482 _]
              tunnel: w478 -> [w481 _]
              frame False {
                n195 = local write "File"(w481) -> ()
                n196 = Enqueue Element(queue=w482, element="Load") -> (queue out=w483:refnum<queue>)  [unwired: 2 in, 2 out]
                n197 = Enqueue Element(queue=w483, element="Renumber") -> ()  [unwired: 2 in, 3 out]
              }
              frame True {
              }
            }
          }
        }
      }
      event "Save": Value Change {
        n198 = event-data() -> ()  [unwired: 1 in, 1 out]
        n199 = Empty String/Path?(string/path="File") -> (empty?=w488:bool)
        n200 = case shown="True" w488 {
          tunnel: [w492 w494] -> w491
          tunnel: "File" -> [w492 _]
          tunnel: [_ w493] -> w486
          frame False {
          }
          frame True {
            n201 = call "File Dialog"() -> ("selected path"=w494:path, "cancelled"=w493:bool)  [unwired: 12 in, 2 out]
          }
        }
        n202 = local read "Script"() -> (w490:string)
        n203 = case shown="False" w486 {
          tunnel: w491 -> [w497 _]
          tunnel: w490 -> [w496 _]
          tunnel: T7."Disabled and Grayed Out" ("Disabled") -> [w495 _]
          frame False {
            n204 = Write to Text File(file (use dialog)=w497, text=w496) -> ()  [unwired: 2 in, 3 out]
            n205 = property on="Save" class="Bool"("DisabledEnum"=w495) -> ()  [unwired: 2 in, 2 out]
          }
          frame True {
          }
        }
      }
      event "View", "Destination", "Color Statistic", "Gray Statistic", "Blob Params", "QR Return", "Params", "Face Parameter": Value Change {
        n206 = event-data() -> ()  [unwired: 1 in, 1 out]
        n207 = call "AddManyToQueue.vi"("Cmds"="Stop\nsimpleView\nRun", "Queue in"=w499) -> ()  [unwired: 9 in, 1 out]
        n208 = local read "Destination"() -> (w500:enum16{"None", "UART", "SPI", "I2C", "WiFi"})
        n209 = local read "View"() -> (w503:T4)
        n210 = To Unsigned Byte Integer(number=w503) -> (unsigned 8bit integer=w502:u8)
        n211 = To Unsigned Byte Integer(number=w500) -> (unsigned 8bit integer=w501:u8)
        n212 = local write "Params"(w502) -> ()
        n213 = local write "Destination Info"(w501) -> ()
      }
      event "Set ROI": Value Change {
        n214 = event-data() -> ()  [unwired: 1 in, 1 out]
        n215 = local read "Tabs"() -> (w504:enum32{"Simple View", "REPL", "Python"})
        n216 = case shown="Default" w504 {
          tunnel: ["Stop\nROI\nsimpleView\nRenumber\nRun" "Stop\nROI\nRun"] -> w505
          frame "Simple View" {
          }
          frame Default {
          }
        }
        n217 = call "AddManyToQueue.vi"("Cmds"=w505, "Queue in"=w506) -> ()  [unwired: 9 in, 1 out]
      }
      event "Plots.L", "Plots.a", "Plots.b": Cursor Move {
        n218 = event-data() -> ()  [unwired: 1 in, 1 out]
        n219 = call "AddManyToQueue.vi"("Cmds"="Stop\nLab\nsimpleView\nRenumber\nRun", "Queue in"=w510) -> ()  [unwired: 9 in, 1 out]
      }
      event "Set Threshold": Value Change {
        n220 = event-data() -> ()  [unwired: 1 in, 1 out]
        n221 = local read "Tabs"() -> (w511:enum32{"Simple View", "REPL", "Python"})
        n222 = case shown="Default" w511 {
          tunnel: ["Stop\nLabPopup\nLab\nsimpleView\nRenumber\nRun" "Stop\nLabPopup\nLab\nRun"] -> w512
          frame "Simple View" {
          }
          frame Default {
          }
        }
        n223 = call "AddManyToQueue.vi"("Cmds"=w512, "Queue in"=w513) -> ()  [unwired: 9 in, 1 out]
      }
      event "clear": Value Change {
        n224 = event-data() -> ()  [unwired: 1 in, 1 out]
        n225 = Enqueue Element(queue=w516, element="Clear") -> ()  [unwired: 2 in, 3 out]
      }
      event "Ctrl C": Value Change {
        n226 = event-data() -> ()  [unwired: 1 in, 1 out]
        n227 = local read "Serial Port"() -> (w519:refnum<visa-resource-name>)
        n228 = VISA Write(VISA resource name=w519, write buffer="\u0003") -> (error out=w518:errorcluster)  [unwired: 1 in, 2 out]
      }
      event "Ctrl D": Value Change {
        n229 = event-data() -> ()  [unwired: 1 in, 1 out]
        n230 = local read "Serial Port"() -> (w522:refnum<visa-resource-name>)
        n231 = VISA Write(VISA resource name=w522, write buffer="\u0004") -> (error out=w521:errorcluster)  [unwired: 1 in, 2 out]
      }
      event "Line": Value Change {
        n232 = event-data() -> ()  [unwired: 1 in, 1 out]
        n233 = property on="Notepad" class="Str"() -> ("Text.Text"=w529:string)  [unwired: 2 in, 2 out]
        n234 = call "Select.vi"("Line"="Line", "Text.Text"=w529) -> ("scale"=w526:i32, "Text min"=w524:i32, "Text max"=w525:i32)  [unwired: 7 in]
        n235 = property on="Line" class="Slide (strict)"("Scale.Maximum"=w526) -> ()  [unwired: 2 in, 2 out]
        n236 = property on="Notepad" class="Str"("Key Focus"=TRUE, "Text.Selection End"=w525, "Text.Selection Start"=w524) -> ()  [unwired: 2 in, 2 out]
      }
      event "Send Line": Value Change {
        n237 = event-data() -> ()  [unwired: 1 in, 1 out]
        n238 = local read "Line"() -> (w532:u8)
        n239 = call "StringToArray.vi"("write buffer"="Notepad") -> ("Array"=w535:string[])  [unwired: 10 in]
        n240 = Index Array(array=w535, index=w532) -> (element=w530:string)
        n241 = call "REPL_Clean.vi"("Code in"=w530) -> ("Code cleaned"=w533:string)  [unwired: 10 in]
        n242 = Enqueue Element(queue=w534, element=w533) -> ()  [unwired: 2 in, 3 out]
        n243 = Increment(x=w532) -> (x+1=w531:u8)
        n244 = property on="Line" class="Slide (strict)"("Val(Sgnl)"=w531) -> ()  [unwired: 2 in, 2 out]
      }
      event "Grab Script": Value Change {
        w537 = u8 0 ("Line")
        n245 = event-data() -> ()  [unwired: 1 in, 1 out]
        n246 = property on="Line" class="Slide (strict)"("Val(Sgnl)"=w537) -> ()  [unwired: 2 in, 2 out]
        n247 = local read "Script"() -> (w538:string)
        n248 = property on="Notepad" class="Str"("Value"=w538, "Text.Scroll Position"=w537) -> ()  [unwired: 2 in, 2 out]
      }
      event "Make Main": Value Change {
        n249 = event-data() -> ()  [unwired: 1 in, 1 out]
        n250 = call "AddManyToQueue.vi"("Cmds"="Stop\nMain.py", "Queue in"=w539) -> ()  [unwired: 9 in, 1 out]
      }
      event Key Down? {
        n251 = event-data() -> ("Char"=w551:i16, "VKey"=w550:T11, "ScanCode"=w549:i16, "Mods"=w548:cluster{"Num Pad":bool, "Menu Key":bool}, "PlatMods"=w547:T12, "FocusObj"=w544:refnum<vi>)  [unwired: 1 in]
        n252 = control-ref of="Console"() -> (w542:refnum<vi>)
        n253 = Bundle("Char"=w551, "VKey"=w550, "ScanCode"=w549, "Mods"=w548, "PlatMods"=w547, "FocusObj"=w544) -> (w543:T13)  [unwired: 1 in]
        n254 = Equal?(x=w544, y=w542) -> (x = y?=w546:bool)
        n255 = case shown="True" w546 {
          tunnel: w543 -> [_ w557]
          tunnel: w545 -> [_ w555]
          tunnel: [_ TRUE] -> w541
          frame False {
          }
          frame True {
            n256 = call "KeyboardCalls.vi"("Cluster"=w557) -> ("Extras"=w553:enum16{"Nix", "clear"}, "string"=w556:string)  [unwired: 9 in]
            n257 = case shown="\"Nix\", Default" w553 {
              tunnel: w555 -> [w558 w561]
              tunnel: [w558 w560] -> w554
              frame "Nix", Default {
              }
              frame "clear" {
                n258 = Enqueue Element(queue=w561, element="cline") -> (queue out=w560:refnum<queue>)  [unwired: 2 in, 2 out]
              }
            }
            n259 = Enqueue Element(queue=w554, element=w556) -> ()  [unwired: 2 in, 3 out]
          }
        }
        n260 = event-data("Discard?"=w541) -> ()  [unwired: 1 in, 1 out]
      }
    }
  }
  n261 = property on="L" class="WFGraph (strict)"("Active Cursor"=u32 0, "Cursor.Cursor X"=10.0 ("Cursor.Cursor Position:Cursor X"), "Active Cursor"=u32 1, "Cursor.Cursor X"=90.0 ("Cursor.Cursor Position:Cursor X")) -> ()  [unwired: 2 in, 2 out]
  n262 = property on="a" class="WFGraph (strict)"("Active Cursor"=u32 0, "Cursor.Cursor X"=-40.0 ("Cursor.Cursor Position:Cursor X"), "Active Cursor"=u32 1, "Cursor.Cursor X"=40.0 ("Cursor.Cursor Position:Cursor X")) -> ()  [unwired: 2 in, 2 out]
  n263 = property on="b" class="WFGraph (strict)"("Active Cursor"=u32 0, "Cursor.Cursor X"=-40.0 ("Cursor.Cursor Position:Cursor X"), "Active Cursor"=u32 1, "Cursor.Cursor X"=40.0 ("Cursor.Cursor Position:Cursor X")) -> ()  [unwired: 2 in, 2 out]
